vi "未命名 3.vi"() -> ()   [LabVIEW 2019]
uses:
  <vilib>/JDP Science/JSONtext/support/Format JSON Object.vi
  <vilib>/addons/Tools/Unicode/UTF8 Tools.lvlib
  <vilib>/JDP Science/JSONtext/JSONtext.lvlib
panel:
  in  "device-list":T1(array[cluster])
  in  "device":T2
  in  "info":T3
  out "数组 3":string[][](array[string])
  in  "pannel-list":T4(array[cluster])=[{"node"=[{"ID"="1", "Attribute"="dev", "Action"="", "name"="台灯"}, {"ID"="2", "Attribute"="dev", "Action"="bright-gear", "name"="阅读灯"}], "ID"="0"}, {"node"=[{"ID"="1", "Attribute"="dev", "Action"="", "name"="顶灯"}, {"ID"="2", "Attribute"="dev", "Action"="", "name"="台灯"}], "ID"="1"}, {"node"=[{"ID"="1", "Attribute"="dev", "Action"="open", "name"="窗帘"}, {"ID"="2", "Attribute"="dev", "Action"="close", "name"="窗帘"}], "ID"="2"}]
  out "<JSON>":string caption="<JSON>Array"
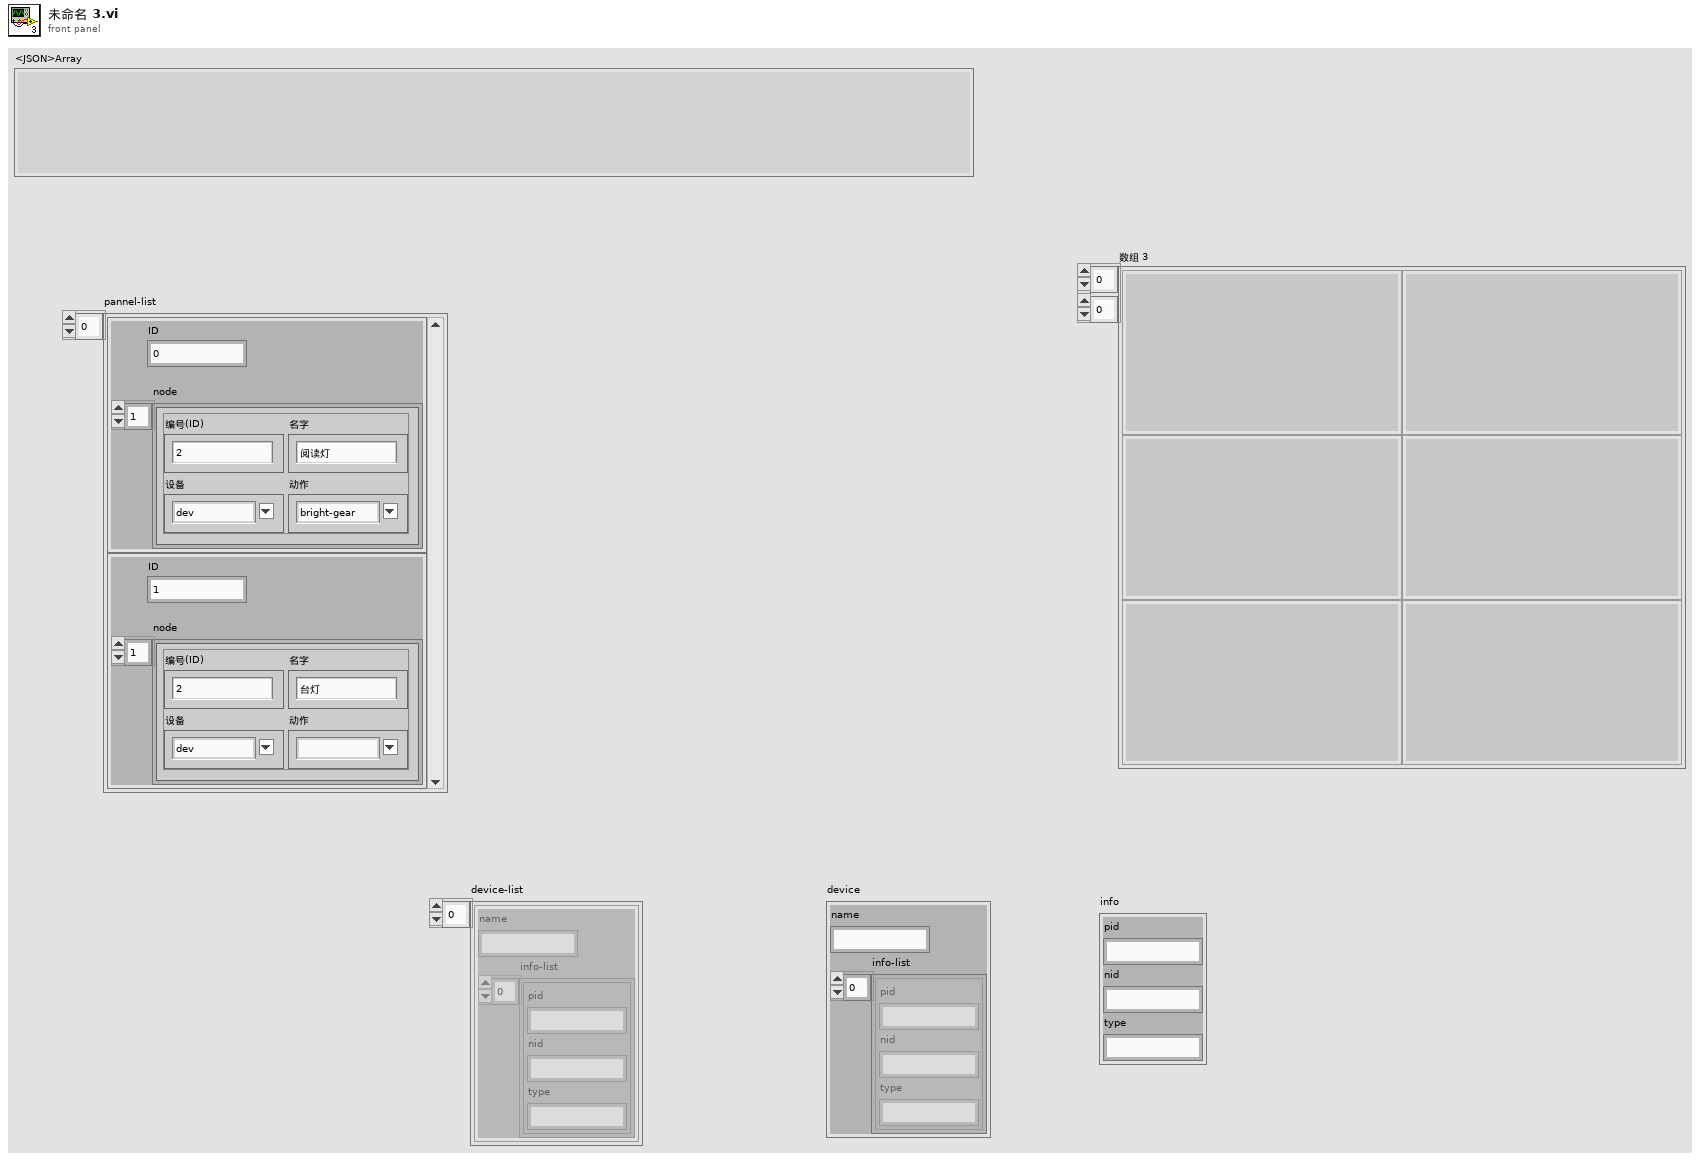
[diagram p1: front panel]
types:
  T1 = cluster{"name":string, "info-list":cluster{"pid":string, "nid":string, "type":string}[]}[]
  T2 = cluster{"name":string, "info-list":cluster{"pid":string, "nid":string, "type":string}[]}
  T3 = cluster{"pid":string, "nid":string, "type":string}
  T4 = cluster{"node":cluster{"ID":string, "Attribute":string, "Action":string, "name":string}[], "ID":string}[]
  T5 = cluster{"ID":string, "Attribute":string, "Action":string, "name":string}[]
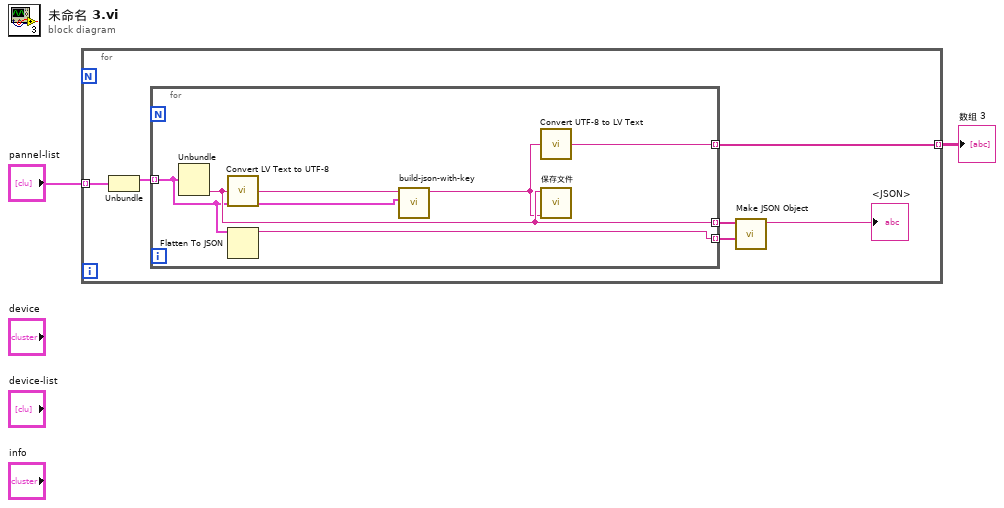
[diagram p0: block diagram]
diagram:
  n1 = for {
    tunnel: "pannel-list" -> [w8] mode=indexing
    tunnel: [w5] -> w1 mode=indexing
    n2 = Unbundle(w8) -> ("node"=w7:T5)  [unwired: 1 out]
    n3 = for {
      tunnel: w7 -> [w12] mode=indexing
      tunnel: [w10] -> w5 mode=indexing
      tunnel: [w13] -> w6 mode=indexing
      tunnel: [w11] -> w3 mode=indexing
      n4 = Unbundle(w12) -> ("name"=w13:string)  [unwired: 3 out]
      n5 = call <vilib>:"Convert LV Text to UTF-8.vi"("LV Text"=w13) -> ("UTF-8 Text"=w14:string)  [unwired: 13 in, 1 out]
      n6 = Flatten To JSON(anything=w12) -> (JSON string=w11:string)  [unwired: 2 in, 1 out]
      n7 = call "build-json-with-key.vi"("value"=w12, "key"=w14) -> ("<JSON>First JSON Value\n\n<JSON>"=w9:string)  [unwired: 9 in]
      n8 = call <vilib>:"Convert UTF-8 to LV Text.vi"("UTF-8 Text"=w9) -> ("LV Text"=w10:string)  [unwired: 13 in, 1 out]
      n9 = call "保存文件.vi"("input"=w9, "文件名"=w13) -> ()  [unwired: 9 in, 1 out]
    }
    n10 = call <vilib>:"Make JSON Object.vi"("JSON Items"=w3, "Item Names"=w6) -> ("<JSON>"=→"<JSON>":string)  [unwired: 8 in, 1 out]
  }
  "数组 3" <- w1
